vi "runtest read cached instruments.vi"(7 "Station":T3, 8 "error in (no error)":errorcluster, 10 "sxSequenceId":string, 11 "Connection Refnum":T1) -> (0 "error out":errorcluster, 2 "Step Associations":T2[](array[typedef]), 3 "Connection Refnum":T1)   [LabVIEW 2011]
uses:
  server/database/Stations/Station Record.ctl
  server/database/Stations/Step Associations/Step Association Record.ctl
  SI.LIB/ODBC/SQL Controls/Connection Refnum.ctl
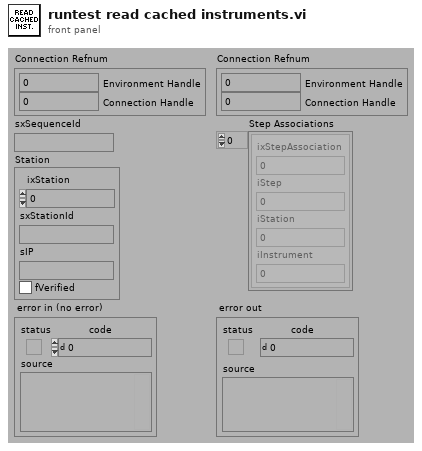
[diagram p1: front panel]
types:
  T1 = typedef "Connection Refnum.ctl" = cluster{"Environment Handle":i32, "Connection Handle":i32}
  T2 = typedef "Step Association Record.ctl" = cluster{"ixStepAssociation":i32, "iStep":i32, "iStation":i32, "iInstrument":i32}
  T3 = typedef "Station Record.ctl" = cluster{"ixStation":i32, "sxStationId":string, "sIP":string, "fVerified":bool}
  T4 = typedef "Step Record.ctl" = cluster{"ixStep":i32, "sxSequenceId":string, "sxTestId":string, "iIndex":i32, "iRepeat":i32, "iQuickMode":i32, "sTag":string, "sDatasheetsCSV":string, "bConfiguration":string}
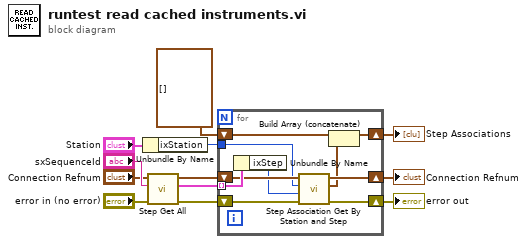
[diagram p0: block diagram]
diagram:
  n1 = Unbundle By Name("Station") -> ("ixStation"=w3:i32)
  n2 = call "Step Get All.vi"("error in (no error)"="error in (no error)", "sxSequenceId"="sxSequenceId", "Connection Refnum"="Connection Refnum") -> ("error out"=w8:errorcluster, "Sequence Steps"=w5:T4[], "Connection Refnum"=w9:T1)  [unwired: 4 in, 2 out]
  n3 = for {
    shift-right: [w20] -> w7
    shift-left: w8 -> [w21]
    shift-right: [w19] -> w6
    shift-left: w9 -> [w18]
    tunnel: w5 -> [w22] mode=indexing
    tunnel: w3 -> [w16]
    shift-right: [w13] -> w1
    shift-left: T2[] [] ("Step Associations") -> [w15]
    n4 = Unbundle By Name(w22) -> ("ixStep"=w17:i32)
    n5 = call "Step Association Get By Station and Step.vi"("error in (no error)"=w21, "iStep (0)"=w17, "iStation (0)"=w16, "Connection Refnum"=w18) -> ("error out"=w20:errorcluster, "Step Associations"=w14:T2[], "Connection Refnum"=w19:T1)  [unwired: 4 in, 1 out]
    n6 = Build Array (concatenate)(w15, w14) -> (w13:T2[])
  }
  "error out" <- w7
  "Step Associations" <- w1
  "Connection Refnum" <- w6
